vi "Open_ESP.vi"(7 "timeout (10sec)":u32=10000, 8 "error in (no error)":errorcluster, 11 "VISA resource name":refnum<visa-resource-name>) -> (0 "error out":errorcluster, 3 "VISA resource name out":refnum<visa-resource-name>)   [LabVIEW 2025]
doc: "Abre la comunicacion con la ESP32\nSe debe colocar siempre al principio de cualquier flujo de programa\nEvitar poner dentro de un ciclo para el correcto funcionamiento"
uses:
  <vilib>/Instr/_visa.llb/VISA Configure Serial Port (Instr).vi
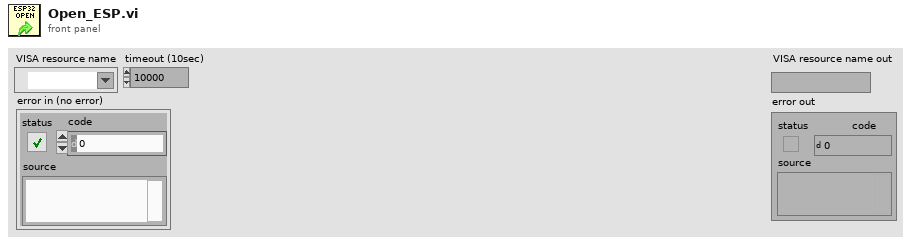
[diagram p1: front panel]
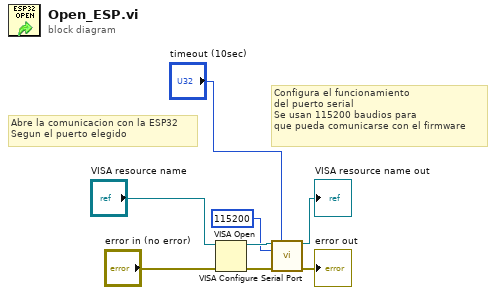
[diagram p0: block diagram]
diagram:
  # "Configura el funcionamiento \ndel puerto serial \nSe usan 115200 baudios para \nque pueda comunicarse con el firmware"
  # "Abre la comunicacion con la ESP32\nSegun el puerto elegido"
  n1 = VISA Open(error in (no error)="error in (no error)", VISA resource name="VISA resource name") -> (VISA resource name=w8:refnum<visa-resource-name>, error out=w7:errorcluster)  [unwired: 3 in]
  n2 = call-poly "VISA Configure Serial Port"("VISA resource name"=w8, "timeout (10sec)"="timeout (10sec)", "baud rate (9600)"=u32 115200, "error in (no error)"=w7) -> ("VISA resource name out"=→"VISA resource name out":refnum<visa-resource-name>, "error out"=→"error out":errorcluster)  [unwired: 10 in]
